vi "Popup.vi"(0 "Back":bool, 11 "Error_In":errorcluster) -> (15 "Error_Out":errorcluster)   [LabVIEW 2021]
doc: "This is Popup VI, which pops-up when the main VI makes it pop-up."
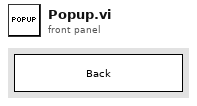
[diagram p1: front panel]
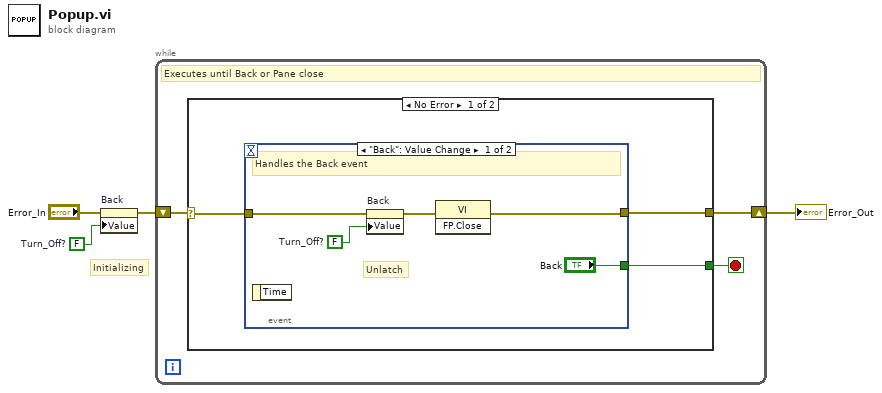
[diagram p0: block diagram]
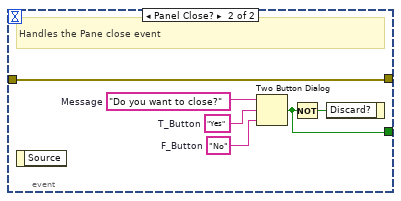
[diagram p2: hidden frame]
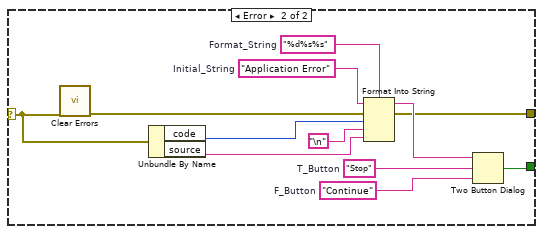
[diagram p3: hidden frame]
diagram:
  w1 = FALSE  # Turn_Off?
  # "Initializing"
  n1 = property on="Back" class="Bool (strict)"(error in="Error_In", "Value"=w1) -> (error out=w2:errorcluster)  [unwired: 1 in, 1 out]
  n2 = while {
    shift-right: [w5] -> w4
    shift-left: w2 -> [w6]
    stop <- w7 stop-if-true
    # "Executes until Back or Pane close"
    n3 = case shown="No Error" w6 {
      selector: w6 -> [w9 w24]
      tunnel: [w10 w22] -> w7
      tunnel: [w8 w23] -> w5
      frame No Error {
        n4 = event shown="[0] \"Back\": Value Change" {
          selector: _ -> [_ _]
          dyn-events: _ -> [_ _]
          timeout: _ -> [_ _]
          tunnel: ["Back" w16] -> w10
          tunnel: w9 -> [w12 w21]
          tunnel: [w14 w21] -> w8
          event "Back": Value Change {
            w11 = FALSE  # Turn_Off?
            # "Unlatch"
            # "Handles the Back event"
            n5 = event-data() -> ()  [unwired: 1 in, 1 out]
            n6 = property on="Back" class="Bool (strict)"(error in=w12, "Value"=w11) -> (error out=w13:errorcluster)  [unwired: 1 in, 1 out]
            n7 = invoke class="VI" method="FP.Close"(error in=w13) -> (error out=w14:errorcluster)  [unwired: 2 in, 2 out]
          }
          event Panel Close? {
            w18 = "Do you want to close?"  # Message
            w19 = "Yes"  # T_Button
            w20 = "No"  # F_Button
            # "Handles the Pane close event"
            n8 = event-data() -> ()  [unwired: 1 in, 1 out]
            n9 = Two Button Dialog(message=w18, 1:w20, 2:w19) -> (T button?=w16:bool)
            n10 = Not(x=w16) -> (.not. x?=w17:bool)
            n11 = event-data("Discard?"=w17) -> ()  [unwired: 1 in, 1 out]
          }
        }
      }
      frame Error {
        w26 = "%d%s%s"  # Format_String
        w27 = "Application Error"  # Initial_String
        w28 = "Stop"  # T_Button
        w29 = "Continue"  # F_Button
        n12 = call <vilib>:"Clear Errors.vi"("error in (no error)"=w24) -> ("error out"=w31:errorcluster)  [unwired: 5 in, 1 out]
        n13 = Unbundle By Name(w24) -> ("code"=w33:i32, "source"=w32:string)
        n14 = Format Into String(format string=w26, initial string=w27, error in=w31, w33, "\n", w32) -> (resulting string=w30:string, error out=w23:errorcluster)
        n15 = Two Button Dialog(message=w30, 1:w29, 2:w28) -> (T button?=w22:bool)
      }
    }
  }
  "Error_Out" <- w4
